vi "Remove Test Folder From lvproj Temporarily.vi"(8 "error in":errorcluster, 11 "custom device path":path) -> (0 "error out":errorcluster, 3 "custom device path out":path)   [LabVIEW 2020, in "Template Tool.lvlib"]
uses:
  Template Tool.lvlib
  Template Tool Global.vi
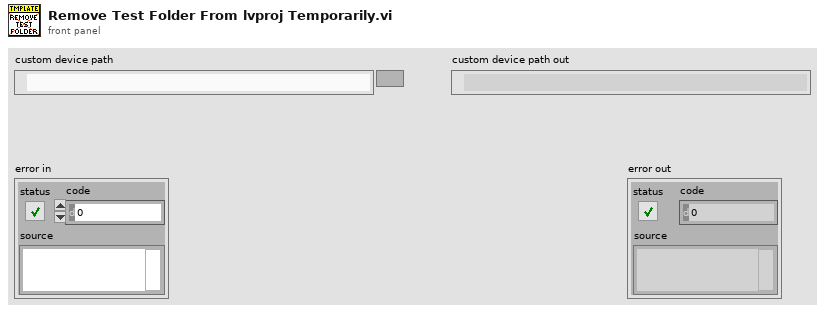
[diagram p1: front panel]
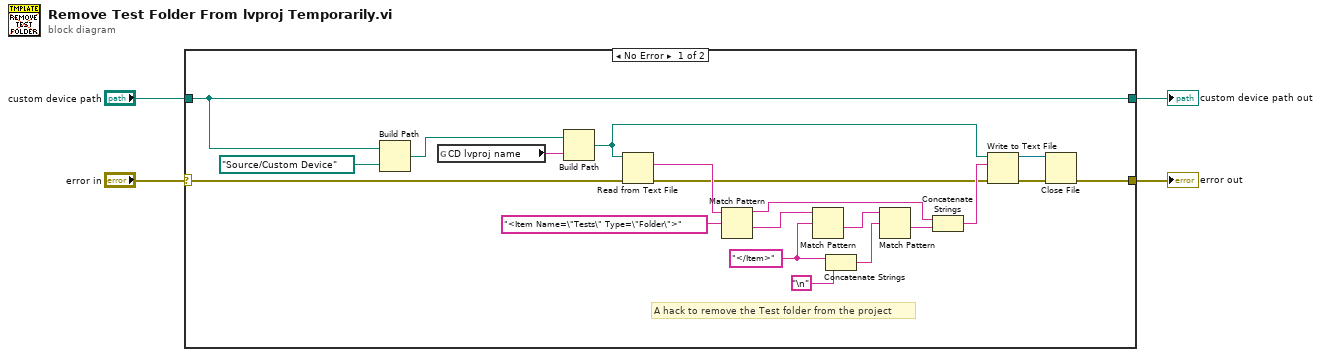
[diagram p0: block diagram]
diagram:
  n1 = case shown="No Error" "error in" {
    selector: "error in" -> [w20 w25]
    tunnel: "custom device path" -> [w19 w26]
    tunnel: [w7 w25] -> w4
    tunnel: [w19 w26] -> w1
    frame No Error {
      w14 = "</Item>" ("regular expression")
      # "A hack to remove the Test folder from the project"
      n2 = Build Path(base path=w19, name or relative path=path "Source/Custom Device") -> (appended path=w23:path)
      n3 = global read "Template Tool Global.vi" "CD lvproj name"() -> (w5:string)
      n4 = Build Path(base path=w23, name or relative path=w5) -> (appended path=w22:path)
      n5 = Read from Text File(file (use dialog)=w22, error in=w20) -> (text=w18:string, error out=w8:errorcluster)  [unwired: 2 in, 2 out]
      n6 = Match Pattern(string=w18, regular expression="<Item Name=\"Tests\" Type=\"Folder\">") -> (before substring=w13:string, after substring=w16:string)  [unwired: 1 in, 2 out]
      n7 = Match Pattern(string=w16, regular expression=w14) -> (after substring=w15:string)  [unwired: 1 in, 3 out]
      n8 = Concatenate Strings(w14, "\n") -> (w11:string)
      n9 = Match Pattern(string=w15, regular expression=w11) -> (after substring=w12:string)  [unwired: 1 in, 3 out]
      n10 = Concatenate Strings(w13, w12) -> (w9:string)
      n11 = Write to Text File(file (use dialog)=w22, text=w9, error in=w8) -> (refnum out=w6:refnum<file>, error out=w21:errorcluster)  [unwired: 1 in, 1 out]
      n12 = Close File(refnum=w6, error in=w21) -> (error out=w7:errorcluster)  [unwired: 1 out]
    }
    frame Error {
    }
  }
  "error out" <- w4
  "custom device path out" <- w1
